vi "sub_create_error_from_body.vi"(7 "error code":i32, 8 "error in (no error)":errorcluster, 10 "http code":i32, 11 "body":string) -> (0 "error out":errorcluster)   [LabVIEW 2013, in "daqio minimal.lvlib"]
doc: "This creates a LabVIEW error from a daq.io server response."
uses:
  daqio minimal.lvlib
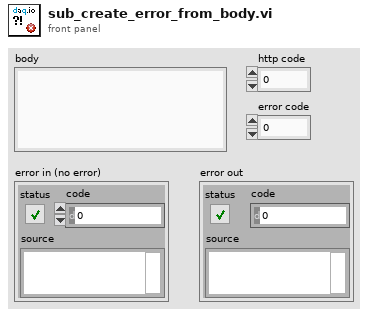
[diagram p1: front panel]
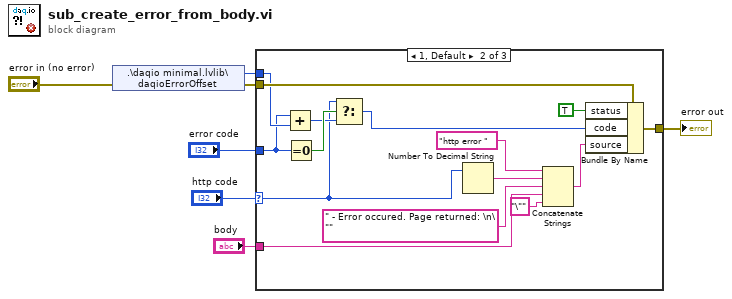
[diagram p0: block diagram]
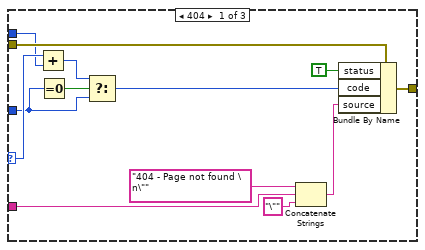
[diagram p2: hidden frame]
diagram:
  n1 = shared-variable ".\\daqio minimal.lvlib\\daqioErrorOffset"(error in="error in (no error)") -> (w1:i32, error out=w2:errorcluster)
  n2 = case shown="1, Default" "http code" {
    selector: "http code" -> [w11 w23 _]
    tunnel: w2 -> [w20 w35 w36]
    tunnel: [w17 w32 w36] -> w7
    tunnel: "body" -> [w14 w29 _]
    tunnel: "error code" -> [w9 w25 _]
    tunnel: w1 -> [w8 w26 _]
    frame 404 {
      n3 = Add(x=w11, y=w8) -> (x+y=w12:i32)
      n4 = Equal To 0?(x=w9) -> (x = 0?=w13:bool)
      n5 = Select(t=w12, s=w13, f=w9) -> (s? t:f=w10:i32)
      n6 = Concatenate Strings("404 - Page not found \n\"" ("string"), w14, "\"" ("string")) -> (w19:string)
      n7 = Bundle By Name(cluster=w20, "status"=TRUE, "code"=w10, "source"=w19) -> (w17:errorcluster)
    }
    frame 1, Default {
      n8 = Add(x=w25, y=w26) -> (x+y=w24:i32)
      n9 = Equal To 0?(x=w25) -> (x = 0?=w28:bool)
      n10 = Select(t=w23, s=w28, f=w24) -> (s? t:f=w27:i32)
      n11 = Number To Decimal String(number=w23) -> (decimal integer string=w22:string)  [unwired: 1 in]
      n12 = Concatenate Strings("http error " ("string"), w22, " - Error occured. Page returned: \n\"" ("string"), w29, "\"" ("string")) -> (w34:string)
      n13 = Bundle By Name(cluster=w35, "status"=TRUE, "code"=w27, "source"=w34) -> (w32:errorcluster)
    }
    frame 100, 200 {
      # "everything went well"
    }
  }
  "error out" <- w7
